vi "Memory.Pointer.Advanced Copy.vi"   [LabVIEW 2016, in "Memory Manager.lvlib" / "Memory.Pointer.lvclass"]
doc: "Moves bytes of data from the <b>src pointer</b> at <b>src offset</b> to the <b>dst pointer</b> at <b>dst offset</b> using the <b>byte order</b> specified. <b>src width</b> and <b>dst width</b> are used to determine how many bytes to move, as well as where the bytes should be read from/written to in memory. For example, to type cast a DBL to a U16, src width would be 8 bytes and dst width would be 2 bytes.\n\nThe optional argument <b>clear dst bytes</b> will clear the subset of bytes within <b>dst pointer</b> before moving data from the <b>src pointer</b>. This is required when type casting from a smaller type to a larger type, as the larger type may have non-zero bytes that will not get overwritten. This argument can be set the FALSE when casting larger types down to smaller types."
uses:
  Memory.Pointer.lvclass
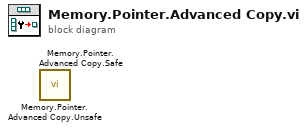
[diagram p0: block diagram]
diagram:
  n1 = call "Memory.Pointer.Advanced Copy.Unsafe.vi"() -> ()  [unwired: 13 in, 3 out]
  n2 = call "Memory.Pointer.Advanced Copy.Safe.vi"() -> ()  [unwired: 13 in, 3 out]
